vi "Interrogate_register.vi"(6 "Address override":i32=-1, 8 "error in (no error)":errorcluster, 9 "UUT Index":i32, 10 "Register mutli-protocol location":T2={"General Parameter name"="", "MODBUS Register"=0, "Profibus"={"Friendly name"="", "PA"={"Slot"=0, "Index"=0}, "DP"={"Slot"=0, "Index"=0}, "Tag"=""}, "Fieldbus"={"Parameter name"="", "Fieldbus Block"="", "Fieldbus Tag"=""}, "data type"=enum."float", "DeviceNET"={"ClassId"=102, "InstanceId"=1, "AttributeId"=12}, "Cluster"={"address"=0, "Mode"=0}, "Length"=0} {"Cluster"."Mode" items=["None", "MODBUS", "HART", "Profibus DP", "Profibus PA", "Fieldbus", "DeviceNET"]}, 11 "MODBUS in":refnum<class "MODBUS.lvclass">) -> (0 "error out":errorcluster, 1 "Parameter name":string, 2 "output":sgl, 3 "MODBUS out":refnum<class "MODBUS.lvclass">, 4 "output cluster":T1)   [LabVIEW 2016, in "MODBUS.lvclass"]
uses:
  MODBUS.lvclass
  Typedef/comm_variable_definition.ctl
  Typedef/Comm_mode_and_address_type.ctl
  Typedef/Comm_mode_type_combo.ctl
  MODBUS.lvclass/MODBUS.ctl
  Protocol Class/Protocol.lvclass
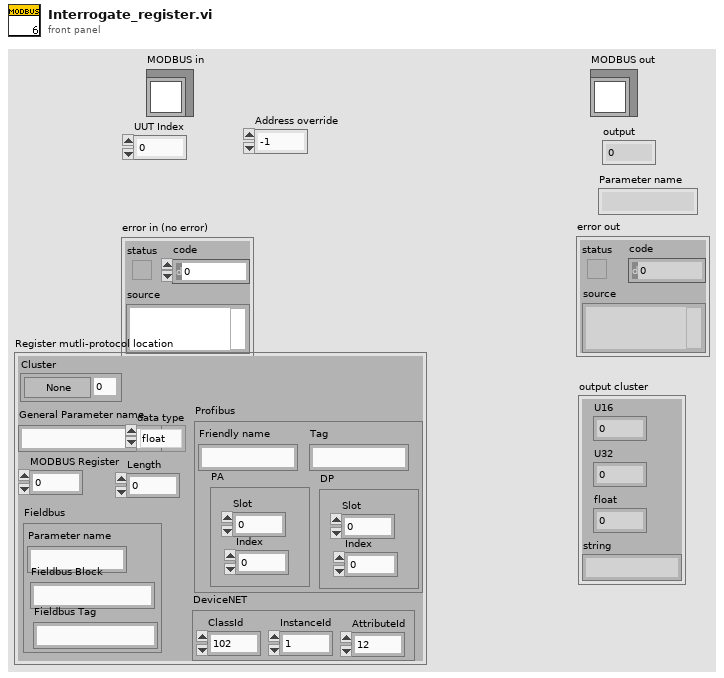
[diagram p1: front panel]
types:
  T1 = cluster{"U16":u16, "U32":u32, "float":sgl, "string":string}
  T2 = typedef "comm_variable_definition.ctl" = cluster{"General Parameter name":string, "MODBUS Register":i32, "Profibus":cluster{"Friendly name":string, "PA":cluster{"Slot":i32, "Index":i32}, "DP":cluster{"Slot":i32, "Index":i32}, "Tag":string}, "Fieldbus":cluster{"Parameter name":string, "Fieldbus Block":string, "Fieldbus Tag":string}, "data type":enum16{"float", "UINT", "UINT32", "STRING"}, "DeviceNET":cluster{"ClassId":u16, "InstanceId":u16, "AttributeId":u8}, "Cluster":T3, "Length":i32}
  T3 = typedef "Comm_mode_and_address_type.ctl" = cluster{"address":i32, "Mode":T4}
  T4 = typedef "Comm_mode_type_combo.ctl" = u16
  T5 = typedef "MODBUS parameters type.ctl" = cluster{"Mode":enum16{"RTU", "ASCII"}, "Default Slave Address":u8, "MODBUS timeout":u32, "Baud Rate":u32, "Parity":u16, "Flow Control":u16}
  T6 = cluster{"Device address":i32, "Switch index":i32}[]
  T7 = cluster{"Device address":i32, "Switch index":i32}
  T8 = enum16{"0-1-2-3", "2-3-0-1", "1-0-3-2", "3-2-1-0"}
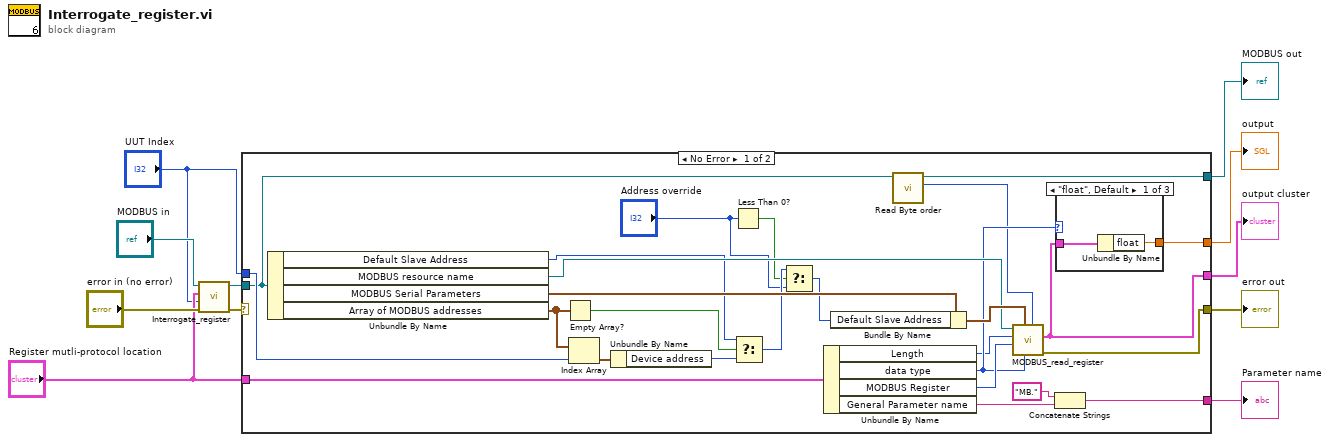
[diagram p0: block diagram]
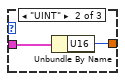
[diagram p2: hidden frame]
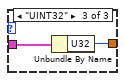
[diagram p3: hidden frame]
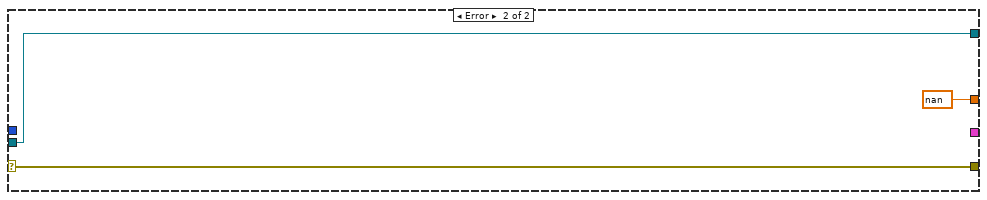
[diagram p4: hidden frame]
diagram:
  n1 = call-parent "Interrogate_register.vi"("error in (no error)"="error in (no error)", "UUT Index"="UUT Index", "Register mutli-protocol location"="Register mutli-protocol location", "Protocol in"="MODBUS in") -> ("error out"=w9:errorcluster, "Protocol out"=w8:refnum<class "MODBUS.lvclass">)  [unwired: 3 in, 3 out]
  n2 = case shown="No Error" w9 {
    selector: w9 -> [_ w46]
    tunnel: "Register mutli-protocol location" -> [w37 _]
    tunnel: [w36 sgl nan ("type single")] -> w3
    tunnel: [w35 w46] -> w4
    tunnel: "UUT Index" -> [w30 _]
    tunnel: w8 -> [w14 w44]
    tunnel: [w12 w44] -> w5
    tunnel: [w26 _] -> w2
    tunnel: [w20 _] -> w1
    frame No Error {
      n3 = Unbundle By Name(w14) -> ("Default Slave Address"=w23:u8, "MODBUS resource name"=w31:refnum<visa-resource-name>, "MODBUS Serial Parameters"=w33:T5, "Array of MODBUS addresses"=w25:T6)
      n4 = Empty Array?(array=w25) -> (empty?=w22:bool)
      n5 = Index Array(array=w25, index=w30) -> (element=w29:T7)
      n6 = Unbundle By Name(w29) -> ("Device address"=w24:i32)
      n7 = Less Than 0?(x="Address override") -> (x < 0?=w17:bool)
      n8 = Select(t=w23, s=w22, f=w24) -> (s? t:f=w18:i32)
      n9 = Select(t=w18, s=w17, f="Address override") -> (s? t:f=w15:i32)
      n10 = Unbundle By Name(w37) -> ("Length"=w19:i32, "data type"=w21:enum16{"float", "UINT", "UINT32", "STRING"}, "MODBUS Register"=w34:i32, "General Parameter name"=w27:string)
      n11 = Bundle By Name(cluster=w33, "Default Slave Address"=w15) -> (w32:T5)
      n12 = call-dynamic "Read Byte order.vi"("Protocol in"=w14) -> ("Byte order"=w13:T8, "Protocol out"=w12:refnum<class "MODBUS.lvclass">)  [unwired: 8 in, 1 out]
      n13 = call "MODBUS_read_register.vi"("Byte order"=w13, "data type"=w21, "MODBUS Serial Parameters"=w32, "Register"=w34, "Length"=w19, "VISA resource name"=w31) -> ("error out"=w35:errorcluster, "output cluster"=w20:T1)  [unwired: 2 in, 2 out]
      n14 = Concatenate Strings("MB." ("Protocol name"), w27) -> (w26:string)
      n15 = case shown="\"float\", Default" w21 {
        tunnel: [w38 w40 w42] -> w36
        tunnel: w20 -> [w39 w41 w43]
        frame "float", Default {
          n16 = Unbundle By Name(w39) -> ("float"=w38:sgl)
        }
        frame "UINT" {
          n17 = Unbundle By Name(w41) -> ("U16"=w40:u16)
        }
        frame "UINT32" {
          n18 = Unbundle By Name(w43) -> ("U32"=w42:u32)
        }
      }
    }
    frame Error {
    }
  }
  "error out" <- w4
  "MODBUS out" <- w5
  "output" <- w3
  "Parameter name" <- w2
  "output cluster" <- w1
